vi "get channels.vi"(11 "OPC UA configuration in":refnum<class "OPC UA Server configuration.lvclass">) -> (2 "channels":refnum<class "TBM channel.lvclass">[](array[class]), 3 "OPC UA configuration out":refnum<class "OPC UA Server configuration.lvclass">)   [LabVIEW 2013, in "OPC UA Server configuration.lvclass"]
uses:
  OPC UA Server configuration.lvclass
  <vilib>/NI/Tag Bus Module Framework/channel/TBM channel.lvclass
  OPC UA Server configuration.lvclass/OPC UA Server configuration.ctl
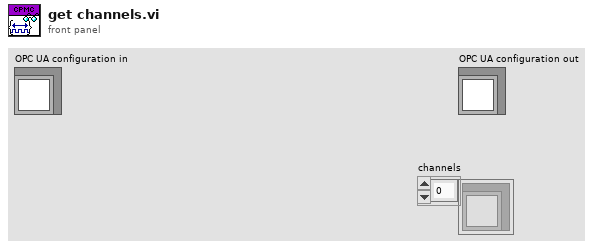
[diagram p1: front panel]
types:
  T1 = typedef "OPC UA Server configuration.lvclass/OPC UA Data Type.ctl" = u16
  T2 = cluster{"channel":refnum<class "TBM channel.lvclass">, "Node Path":string, "OPC UA Data Type":T1}[]
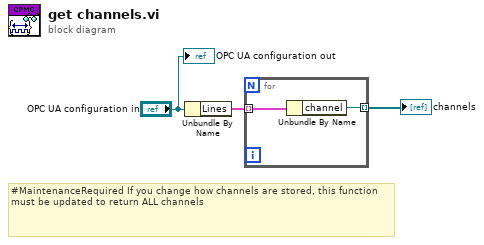
[diagram p0: block diagram]
diagram:
  # "#MaintenanceRequired If you change how channels are stored, this function must be updated to return ALL channels"
  n1 = Unbundle By Name("OPC UA configuration in") -> ("Lines"=w2:T2)
  n2 = for {
    tunnel: w2 -> [w5] mode=indexing
    tunnel: [w4] -> w1 mode=indexing
    n3 = Unbundle By Name(w5) -> ("channel"=w4:refnum<class "TBM channel.lvclass">)
  }
  "channels" <- w1
  "OPC UA configuration out" <- "OPC UA configuration in"
